vi "Dynamic Headers Read Header File.vi"(5 "Tree Selection":T1="Select Room/Stall", 6 "Read/Write (True/False)":bool, 7 "New Header Save Array Write":T3[](array[typedef]), 8 "Error In":errorcluster, 9 "Point Data":T2[](array[typedef]), 10 "Save Data (READ ONLY)":string[][](array[string]), 11 "Tool Base Path":path) -> (0 "Error Out":errorcluster, 3 "New Header Save Array (READ ONLY)":T3[](array[typedef]))   [LabVIEW 2019]
uses:
  Washer DOE/Type Definitions/DOE Data Save Modifier.ctl
  Refrigeration/RTS/Type Definitions/RTS Point File.ctl
  Refrigeration/RTS/Type Definitions/RTS Room Selector.ctl
  <vilib>/Utility/file.llb/Write Delimited Spreadsheet (string).vi
  <vilib>/Utility/file.llb/Read Delimited Spreadsheet (string).vi
panel:
  out "Numeric":i32
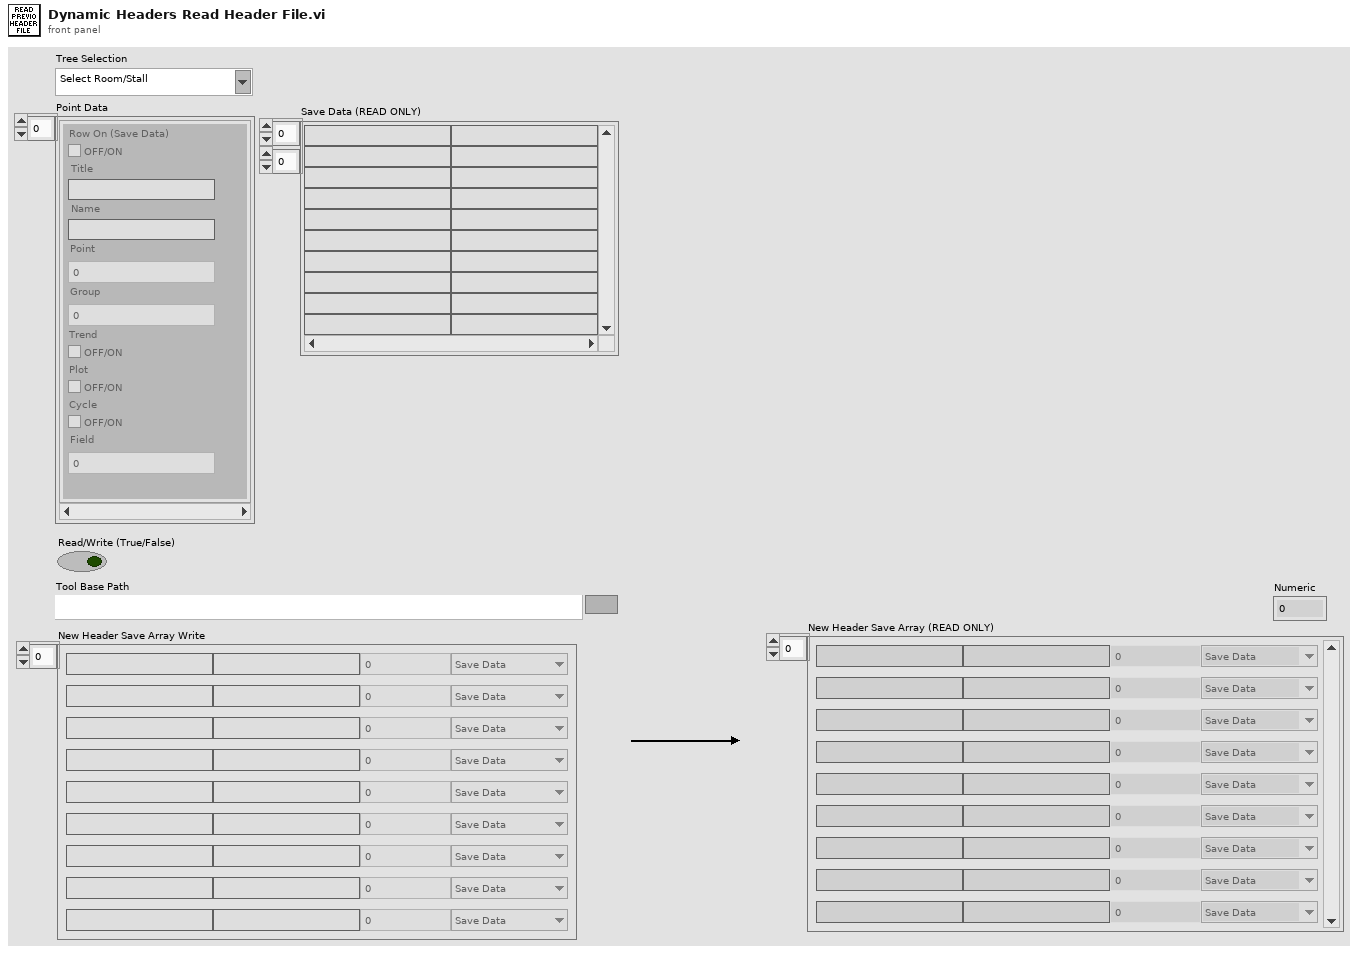
[diagram p1: front panel]
types:
  T1 = typedef "RTS Room Selector.ctl" = string
  T2 = typedef "RTS Point File.ctl" = cluster{"Title":string, "Name":string, "Point":u8, "Plot":bool, "Trend":bool, "Cycle":bool, "Field":u8, "Row On (Save Data)":bool, "Group":u8}
  T3 = typedef "DOE Data Save Modifier.ctl" = cluster{"Name":string, "Title":string, "Save Status":enum16{"Save Data", "Don't Save Data"}, "Group":u8, "Field":u8}
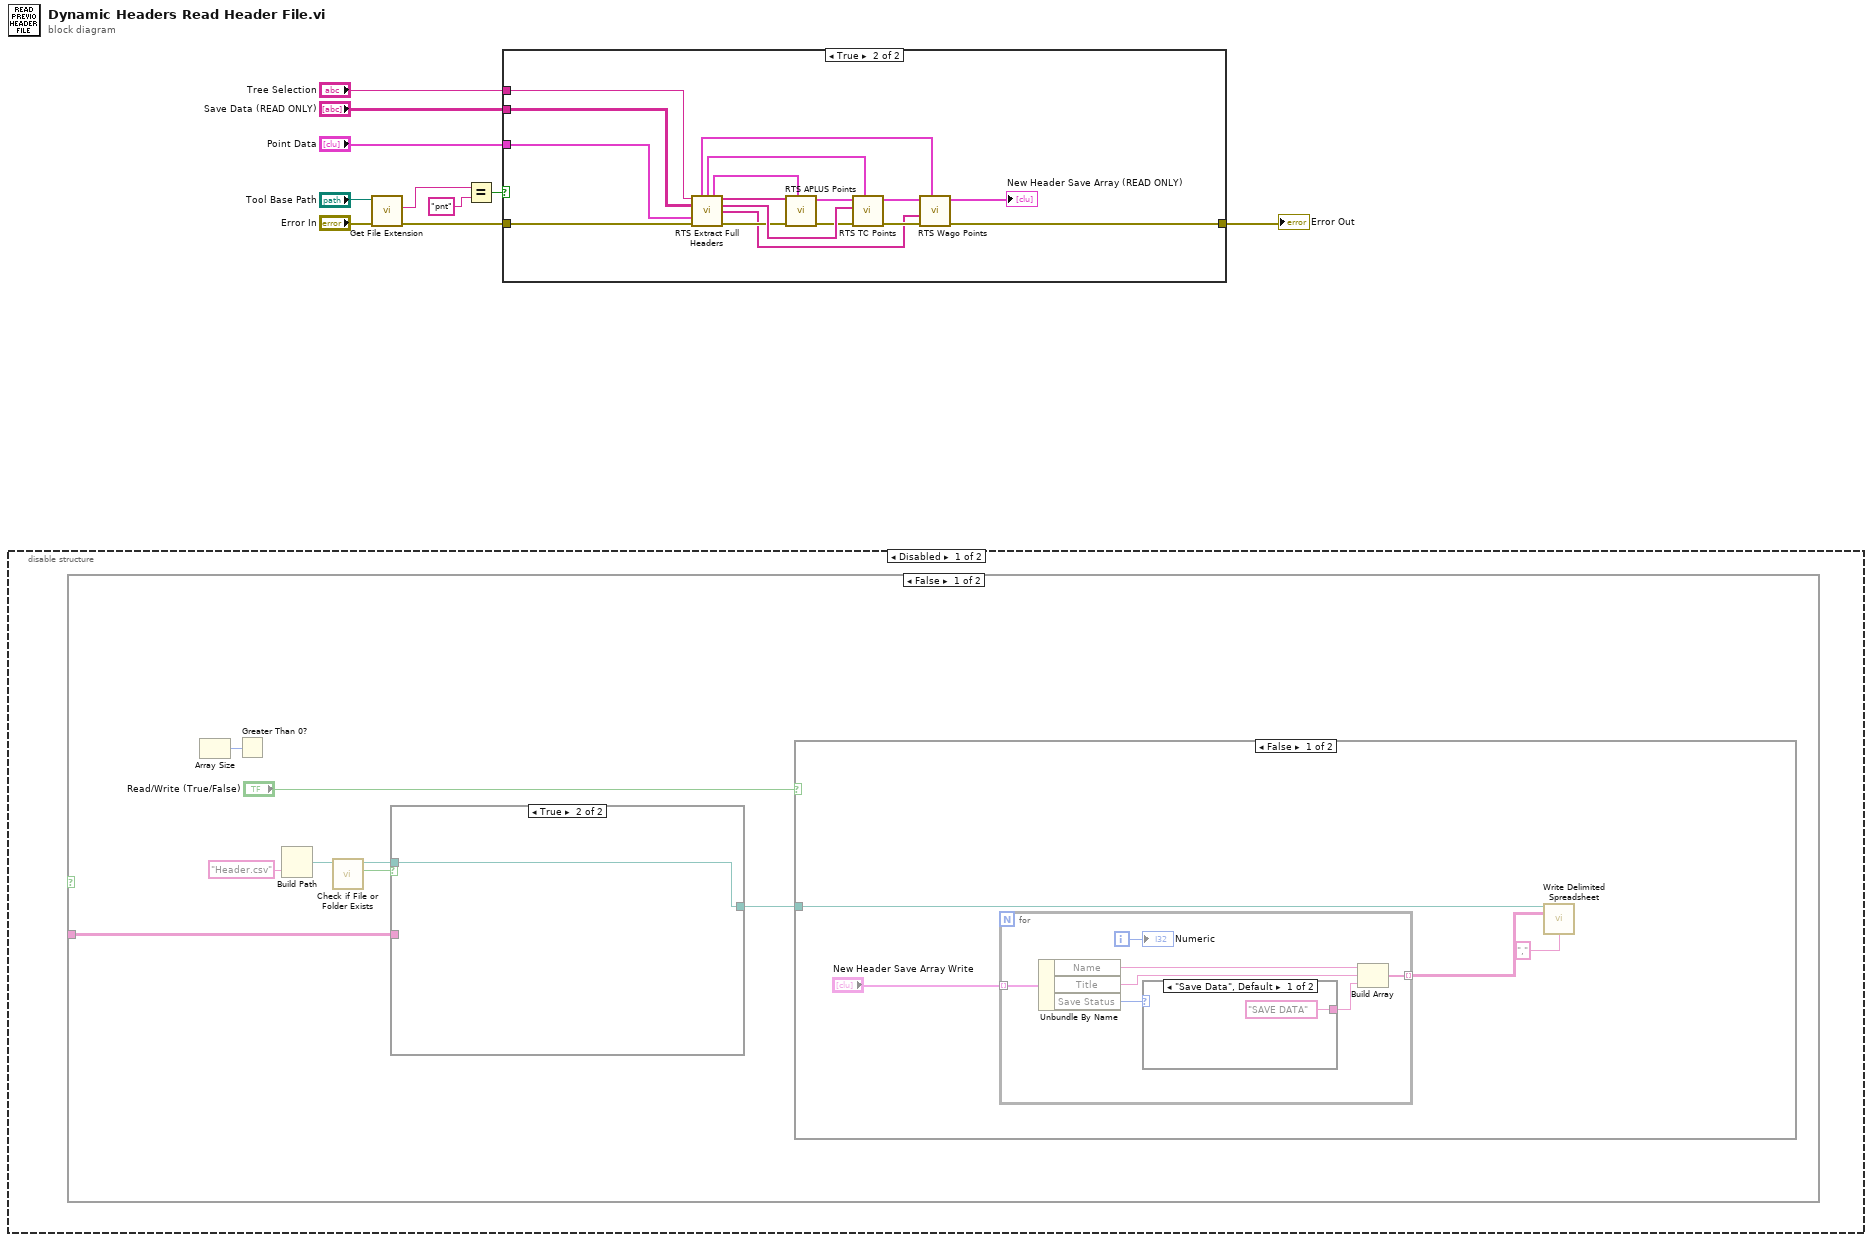
[diagram p0: block diagram]
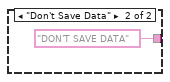
[diagram p2: hidden frame]
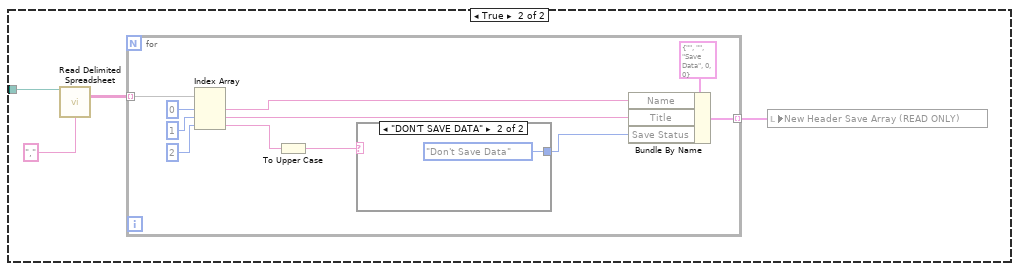
[diagram p3: hidden frame]
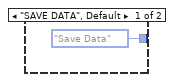
[diagram p4: hidden frame]
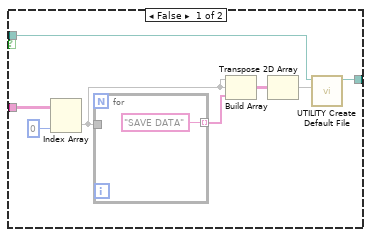
[diagram p5: hidden frame]
diagram:
  n1 = disable-structure shown="Disabled" {
    frame Disabled {
      n2 = case shown="False" {
        selector: _ -> [_ _]
        tunnel: _ -> [w12 _]
        frame False {
          n3 = Array Size() -> (size(s)=w11:i32)  [unwired: 1 in]
          n4 = Greater Than 0?(x=w11) -> ()  [unwired: 1 out]
          n5 = Build Path(name or relative path="Header.csv") -> (appended path=w16:path)  [unwired: 1 in]
          n6 = call <vilib>:"Check if File or Folder Exists.vi"("path"=w16) -> ("file or folder exists?"=w18:bool, "dup path"=w17:path)  [unwired: 8 in, 1 out]
          n7 = case shown="True" w18 {
            tunnel: w17 -> [w51 w58]
            tunnel: [w50 w58] -> w14
            tunnel: w12 -> [w49 _]
            frame False {
              n8 = Index Array(array=w49, index (col)=0 ("disabled index (col)")) -> (element=w55)  [unwired: 1 in]
              n9 = for {
                tunnel: w55 -> [_]
                tunnel: ["SAVE DATA"] -> w56 mode=indexing
              }
              n10 = Build Array(w55, w55, w56) -> (w54:string[][])
              n11 = Transpose 2D Array(2D array=w54) -> (transposed array=w52:string[][])
              n12 = call "UTILITY Create Default File.vi"("Default File"=w52, "Initial DOE Config"=w51) -> ("new file path (Not A Path if cancelled)"=w50:path)  [unwired: 8 in, 1 out]
            }
            frame True {
            }
          }
          n13 = case shown="False" "Read/Write (True/False)" {
            tunnel: w14 -> [w20 w33]
            frame False {
              n14 = for {
                tunnel: "New Header Save Array Write" -> [w29] mode=indexing
                tunnel: [w24] -> w22 mode=indexing
                i -> [w23]
                n15 = Unbundle By Name(w29) -> ("Name"=w27:string, "Title"=w26:string, "Save Status"=w28:enum16{"Save Data", "Don't Save Data"})
                n16 = case shown="\"Save Data\", Default" w28 {
                  tunnel: ["SAVE DATA" "DON'T SAVE DATA"] -> w25
                  frame "Save Data", Default {
                  }
                  frame "Don't Save Data" {
                  }
                }
                n17 = Build Array(w27, w26, w25) -> (w24:string[])
                "Numeric" <- w23
              }
              n18 = call-poly <vilib>:"Write Delimited Spreadsheet.vi"("file path (dialog if empty)"=w20, "2D data"=w22, "delimiter (\\t)"="," ("delimiter (\\t)")) -> ()  [unwired: 11 in, 2 out]
            }
            frame True {
              n19 = call-poly <vilib>:"Read Delimited Spreadsheet.vi"("file path (dialog if empty)"=w33, "delimiter (\\t)"="," ("delimiter (\\t)")) -> ("all rows"=w35:string[][])  [unwired: 8 in, 5 out]
              n20 = for {
                tunnel: w35 -> [w46] mode=indexing
                tunnel: [w36] -> w32 mode=indexing
                n21 = Index Array(array=w46, index #1=0 ("index"), index #2=1 ("index"), index #3=2 ("index")) -> (element #1=w41:string, element #2=w40:string, element #3=w39:string)
                n22 = To Upper Case(1:w39) -> (0:w38:string)
                n23 = case shown="\"DON'T SAVE DATA\"" w38 {
                  tunnel: [enum16{"Save Data", "Don't Save Data"}."Save Data" ("Save Status") enum16{"Save Data", "Don't Save Data"}."Don't Save Data" ("Save Status")] -> w37
                  frame "SAVE DATA", Default {
                  }
                  frame "DON'T SAVE DATA" {
                  }
                }
                n24 = Bundle By Name(cluster=T3 {"Name"="", "Title"="", "Save Status"=enum."Save Data", "Group"=0, "Field"=0} ("Cluster"), "Name"=w41, "Title"=w40, "Save Status"=w37) -> (w36:T3)
              }
              n25 = local write "New Header Save Array (READ ONLY)"(w32) -> ()
            }
          }
        }
        frame True {
        }
      }
    }
    frame Enabled {
    }
  }
  n26 = call <vilib>:"Get File Extension.vi"("error in (no error)"="Error In", "file"="Tool Base Path") -> ("error out"=w2:errorcluster, "lowercase file extension"=w8:string)  [unwired: 5 in, 3 out]
  n27 = Equal?(x=w8, y="pnt") -> (x = y?=w6:bool)
  n28 = case shown="True" w6 {
    tunnel: "Save Data (READ ONLY)" -> [_ w75]
    tunnel: "Tree Selection" -> [_ w76]
    tunnel: "Point Data" -> [_ w66]
    tunnel: w2 -> [w59 w64]
    tunnel: [w59 w60] -> w1
    frame False {
    }
    frame True {
      n29 = call "RTS Extract Full Headers.vi"("Tree Selection in"=w76, "Chamber Data"=w75, "Point Data"=w66, "Error In"=w64) -> ("Wago Point Data"=w61:T2[], "TC Point Data"=w62:T2[], "APLUS Point Data"=w63:T2[], "APLUS Data"=w71:string[], "TC Data"=w74:string[], "Wago Data"=w65:string[], "Error Out"=w73:errorcluster)  [unwired: 5 in]
      n30 = call "RTS APLUS Points.vi"("Point Data"=w63, "Error In"=w73, "APLUS Data"=w71) -> ("Error Out"=w72:errorcluster, "APLUS Data"=w69:T3[])  [unwired: 7 in]
      n31 = call "RTS TC Points.vi"("Point Data"=w62, "Error In"=w72, "TC Data"=w74, "Input Save Array"=w69) -> ("Error Out"=w70:errorcluster, "Output Save Array"=w68:T3[])  [unwired: 6 in]
      n32 = call "RTS Wago Points.vi"("Point Data"=w61, "Error In"=w70, "Wago Data"=w65, "Input Save Array"=w68) -> ("Error Out"=w60:errorcluster, "Output Save Array"=→"New Header Save Array (READ ONLY)":T3[])  [unwired: 6 in]
    }
  }
  "Error Out" <- w1
